vi "database_connection_write_dev_MQTT_no_database_array.vi"(6 "connection reference":T2, 7 "string":string="Raw.DMG_MORI_DMU_40_EVO", 8 "error in (no error)":errorcluster, 9 "data 2":dbl[](array[numeric]), 10 "Machine Data":T3={"Zload"="", "Yload"="", "Xload"="", "path_position"="", "Fovr"="", "SspeedOvr"="", "Program Name"="", "Program status"="", "Block of code being executed"="", "Line of code"="", "Machine availability"="", "Emergency status"="", "Controller mode"="", "Tool_id"="UNAVAILABLE"}, 11 "current time 2":timestamp format="%^<%Y-%m-%d %H:%M:%S%3u>T") -> (0 "connection reference out":T2, 3 "error out":errorcluster)   [LabVIEW 2017]
uses:
  <vilib>/addons/database/Connection.llb/Conn ObjectReference.ctl
  data_base_structure_V2.ctl
  data_base_structure.ctl
  controls/databse_structure.ctl
  <vilib>/addons/database/NI_Database_API.lvlib
panel:
  out "output cluster 2":cluster{string, "Machine availability":string}
  out "output cluster":T1
  out "Array":string[](array[string])=["timestamp", "available", "execution", "controller_mode", "spindle_load", "spindle_speed", "sspeedovr", "feed_rate", "fovr", "I_part", "J_part", "K_part", "Xpos_part", "Ypos_part", "Zpos_part", "Apos_machine", "Bpos_machine", "Xload", "Yload", "Zload", "Aload", "Bload", "tool_id", "program_number", "program_name", "block_code", "line_number", "estop", "accel_x_rms", "accel_y_rms", "accel_z_rms"]
  out "Program Name":string
  out "date/time string 2":string
  out "ISO-8601 UTC Formatted DateTime String":string
  out "error out 2":errorcluster
  in  "error in":errorcluster
  out "Timestamp":timestamp
  out "date/time string":string
  out "current time 3":timestamp
  out "resulting string 2":string
  out "Xload":string
  out "Machine availability":string
  out "resulting string":string
  out "output array 2":dbl[](array[numeric])
  out "size(s) 2":i32
  out "valueSent 2":string="14:19:17.238_"
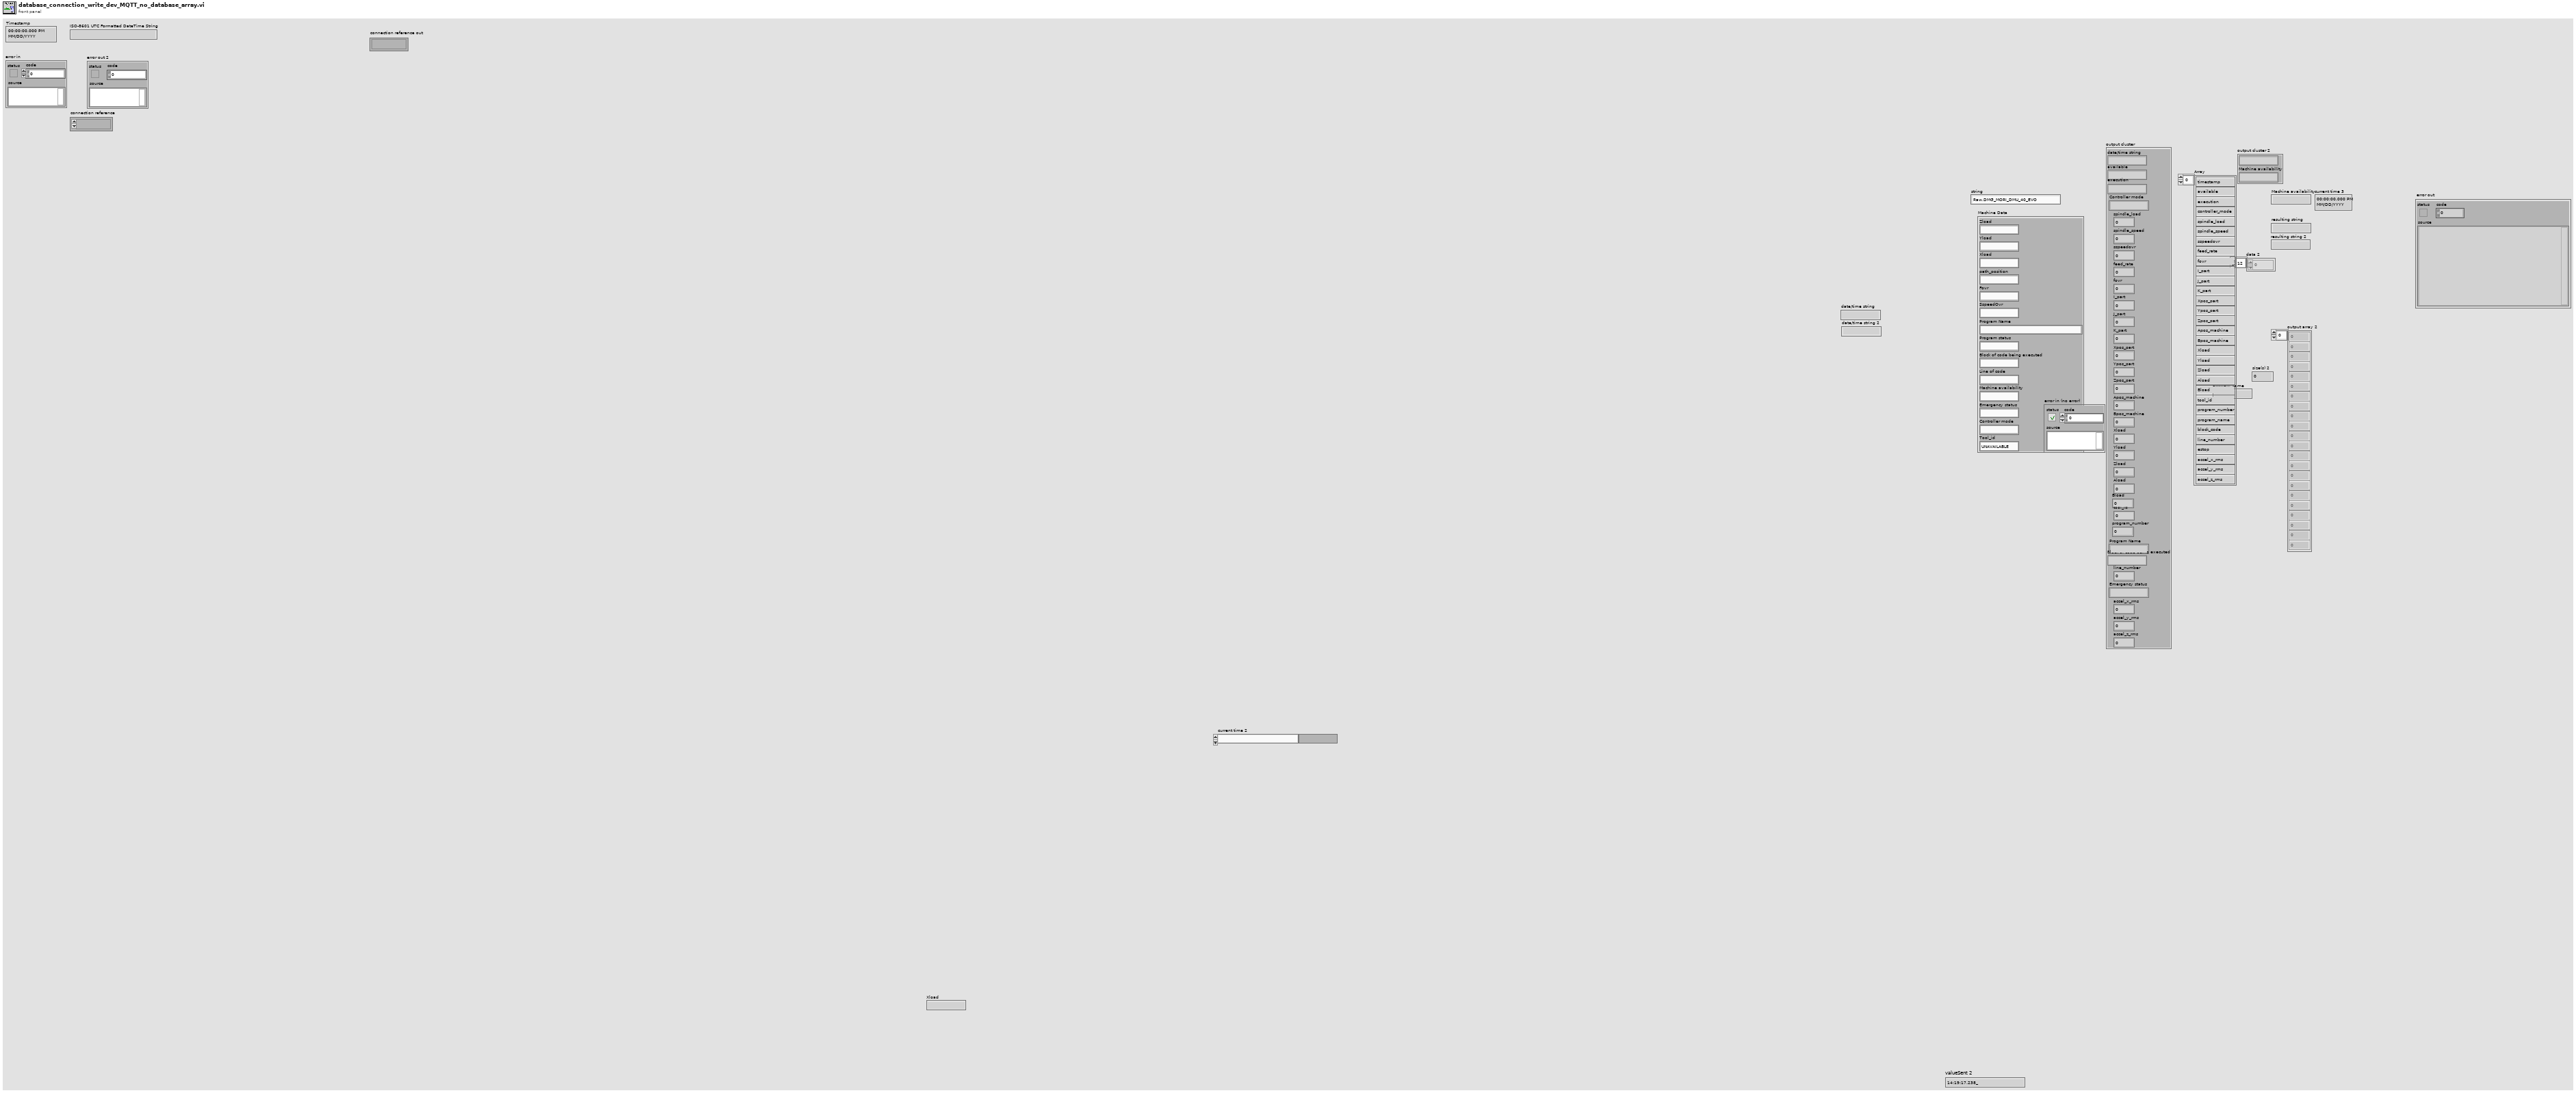
[diagram p1: front panel]
types:
  T1 = typedef "data_base_structure_V2.ctl" = cluster{"date/time string":string, "available":string, "Controller mode":string, "spindle_load":dbl, "spindle_speed":dbl, "sspeedovr":dbl, "feed_rate":dbl, "fovr":dbl, "I_part":dbl, "J_part":dbl, "K_part":dbl, "Xpos_part":dbl, "Ypos_part":dbl, "Zpos_part":dbl, "Apos_machine":dbl, "Bpos_machine":dbl, "Xload":dbl, "Yload":dbl, "Zload":dbl, "Aload":dbl, "Bload":dbl, "tool_id":dbl, "program_number":dbl, "Program Name":string, "Block of code being executed":string, "line_number":dbl, "Emergency status":string, "accel_x_rms":dbl, "accel_y_rms":dbl, "accel_z_rms":dbl, "execution":string}
  T2 = typedef "NI_Database_API.lvlib/Conn ObjectReference.ctl" = refnum<k1>
  T3 = cluster{"Zload":string, "Yload":string, "Xload":string, "path_position":string, "Fovr":string, "SspeedOvr":string, "Program Name":string, "Program status":string, "Block of code being executed":string, "Line of code":string, "Machine availability":string, "Emergency status":string, "Controller mode":string, "Tool_id":string}
  T4 = typedef "data_base_structure.ctl" = cluster{"available ":dbl, "controller_mode":string, "spindle_load":dbl, "spindle_speed ":dbl, "sspeedovr":dbl, "J_part":dbl, "K_part":dbl, "Xpos_part":dbl, "Ypos_part":dbl, "Zpos_part":dbl, "Apos_machine":dbl, "Bpos_machine":dbl, "Xload":dbl, "Yload":dbl, "Zload":dbl, "Aload":dbl, "Bload":dbl, "tool_id":dbl, "program_name":string, "block_code":string, "line_number":dbl, "estop":string, "accel_x_rms":dbl, "accel_y_rms":dbl, "accel_z_rms":dbl, "program_number":dbl, "timestamp":string, "feed_rate ":dbl, "fovr":dbl, "I_part ":dbl}
  T5 = cluster{"date/time string":string, "available":string, "execution":string, "Controller mode":string, "spindle_load":dbl, "spindle_speed":dbl, "sspeedovr":dbl, "feed_rate":dbl, "fovr":dbl, "I_part":dbl, "J_part":dbl, "K_part":dbl, "Xpos_part":dbl, "Ypos_part":dbl, "Zpos_part":dbl, "Apos_machine":dbl, "Bpos_machine":dbl, "Xload":dbl, "Yload":dbl, "Zload":dbl, "Aload":dbl, "Bload":dbl, "tool_id":dbl, "program_number":dbl, "Program Name":string, "Block of code being executed":string, "line_number":dbl, "Emergency status":string, "accel_x_rms":dbl, "accel_y_rms":dbl, "accel_z_rms":dbl}
  T6 = typedef "databse_structure.ctl" = cluster{"date/time string":string, "available":string, "execution":string, "Controller mode":string, "accel_z_rms":dbl, "accel_y_rms":dbl, "accel_x_rms":dbl, "Emergency status":string, "line_number":dbl, "Block of code being executed":string, "Program Name":string, "program_number":dbl, "tool_id":dbl, "Bload":dbl, "Aload":dbl, "Zload":dbl, "Yload":dbl, "Xload":dbl, "Bpos_machine":dbl, "Apos_machine":dbl, "Zpos_part":dbl, "Ypos_part":dbl, "Xpos_part":dbl, "K_part":dbl, "J_part":dbl, "I_part":dbl, "fovr":dbl, "feed_rate":dbl, "sspeedovr":dbl, "spindle_speed":dbl, "spindle_load":dbl}
  T7 = cluster{"data 2[0]":dbl, "data 2[1]":dbl, "data 2[2]":dbl, "data 2[3]":dbl, "data 2[4]":dbl, "data 2[5]":dbl, "data 2[6]":dbl, "data 2[7]":dbl, "data 2[8]":dbl, "data 2[9]":dbl, "data 2[10]":dbl, "data 2[11]":dbl, "data 2[12]":dbl, "data 2[13]":dbl, "data 2[14]":dbl, "data 2[15]":dbl, "data 2[16]":dbl, "data 2[17]":dbl, "data 2[18]":dbl, "data 2[19]":dbl, "data 2[20]":dbl, "data 2[21]":dbl}
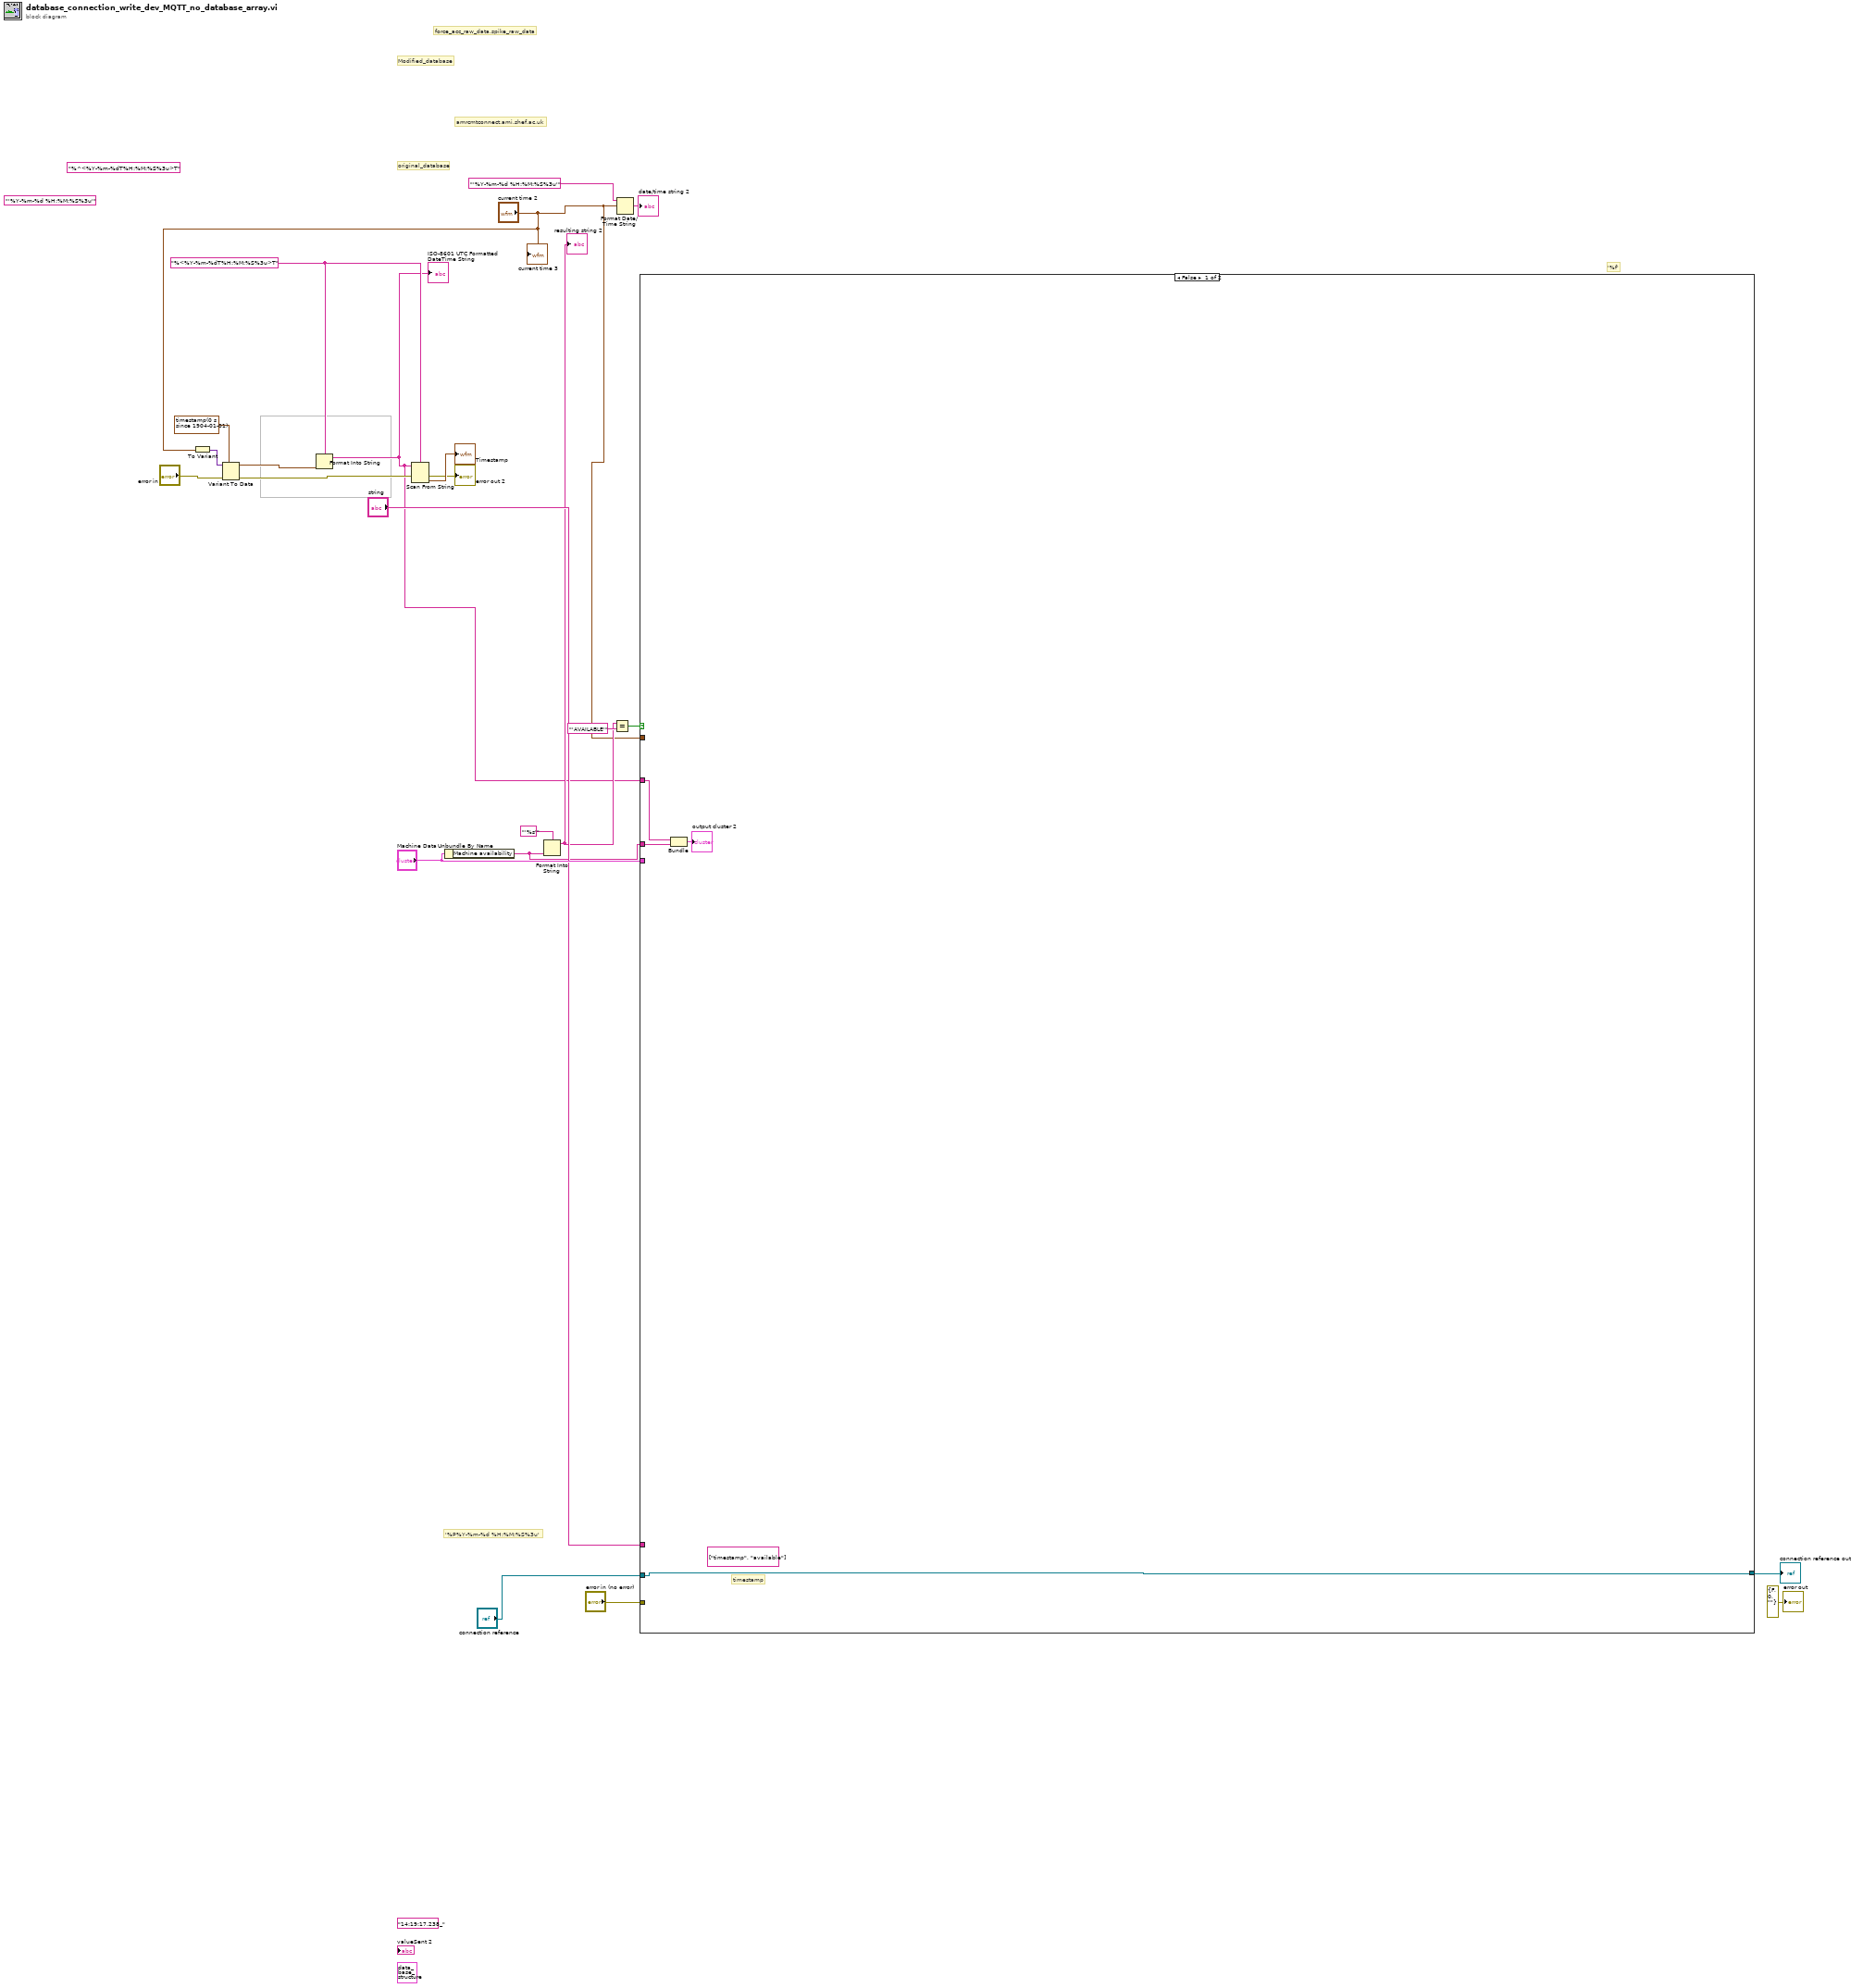
[diagram p0: block diagram]
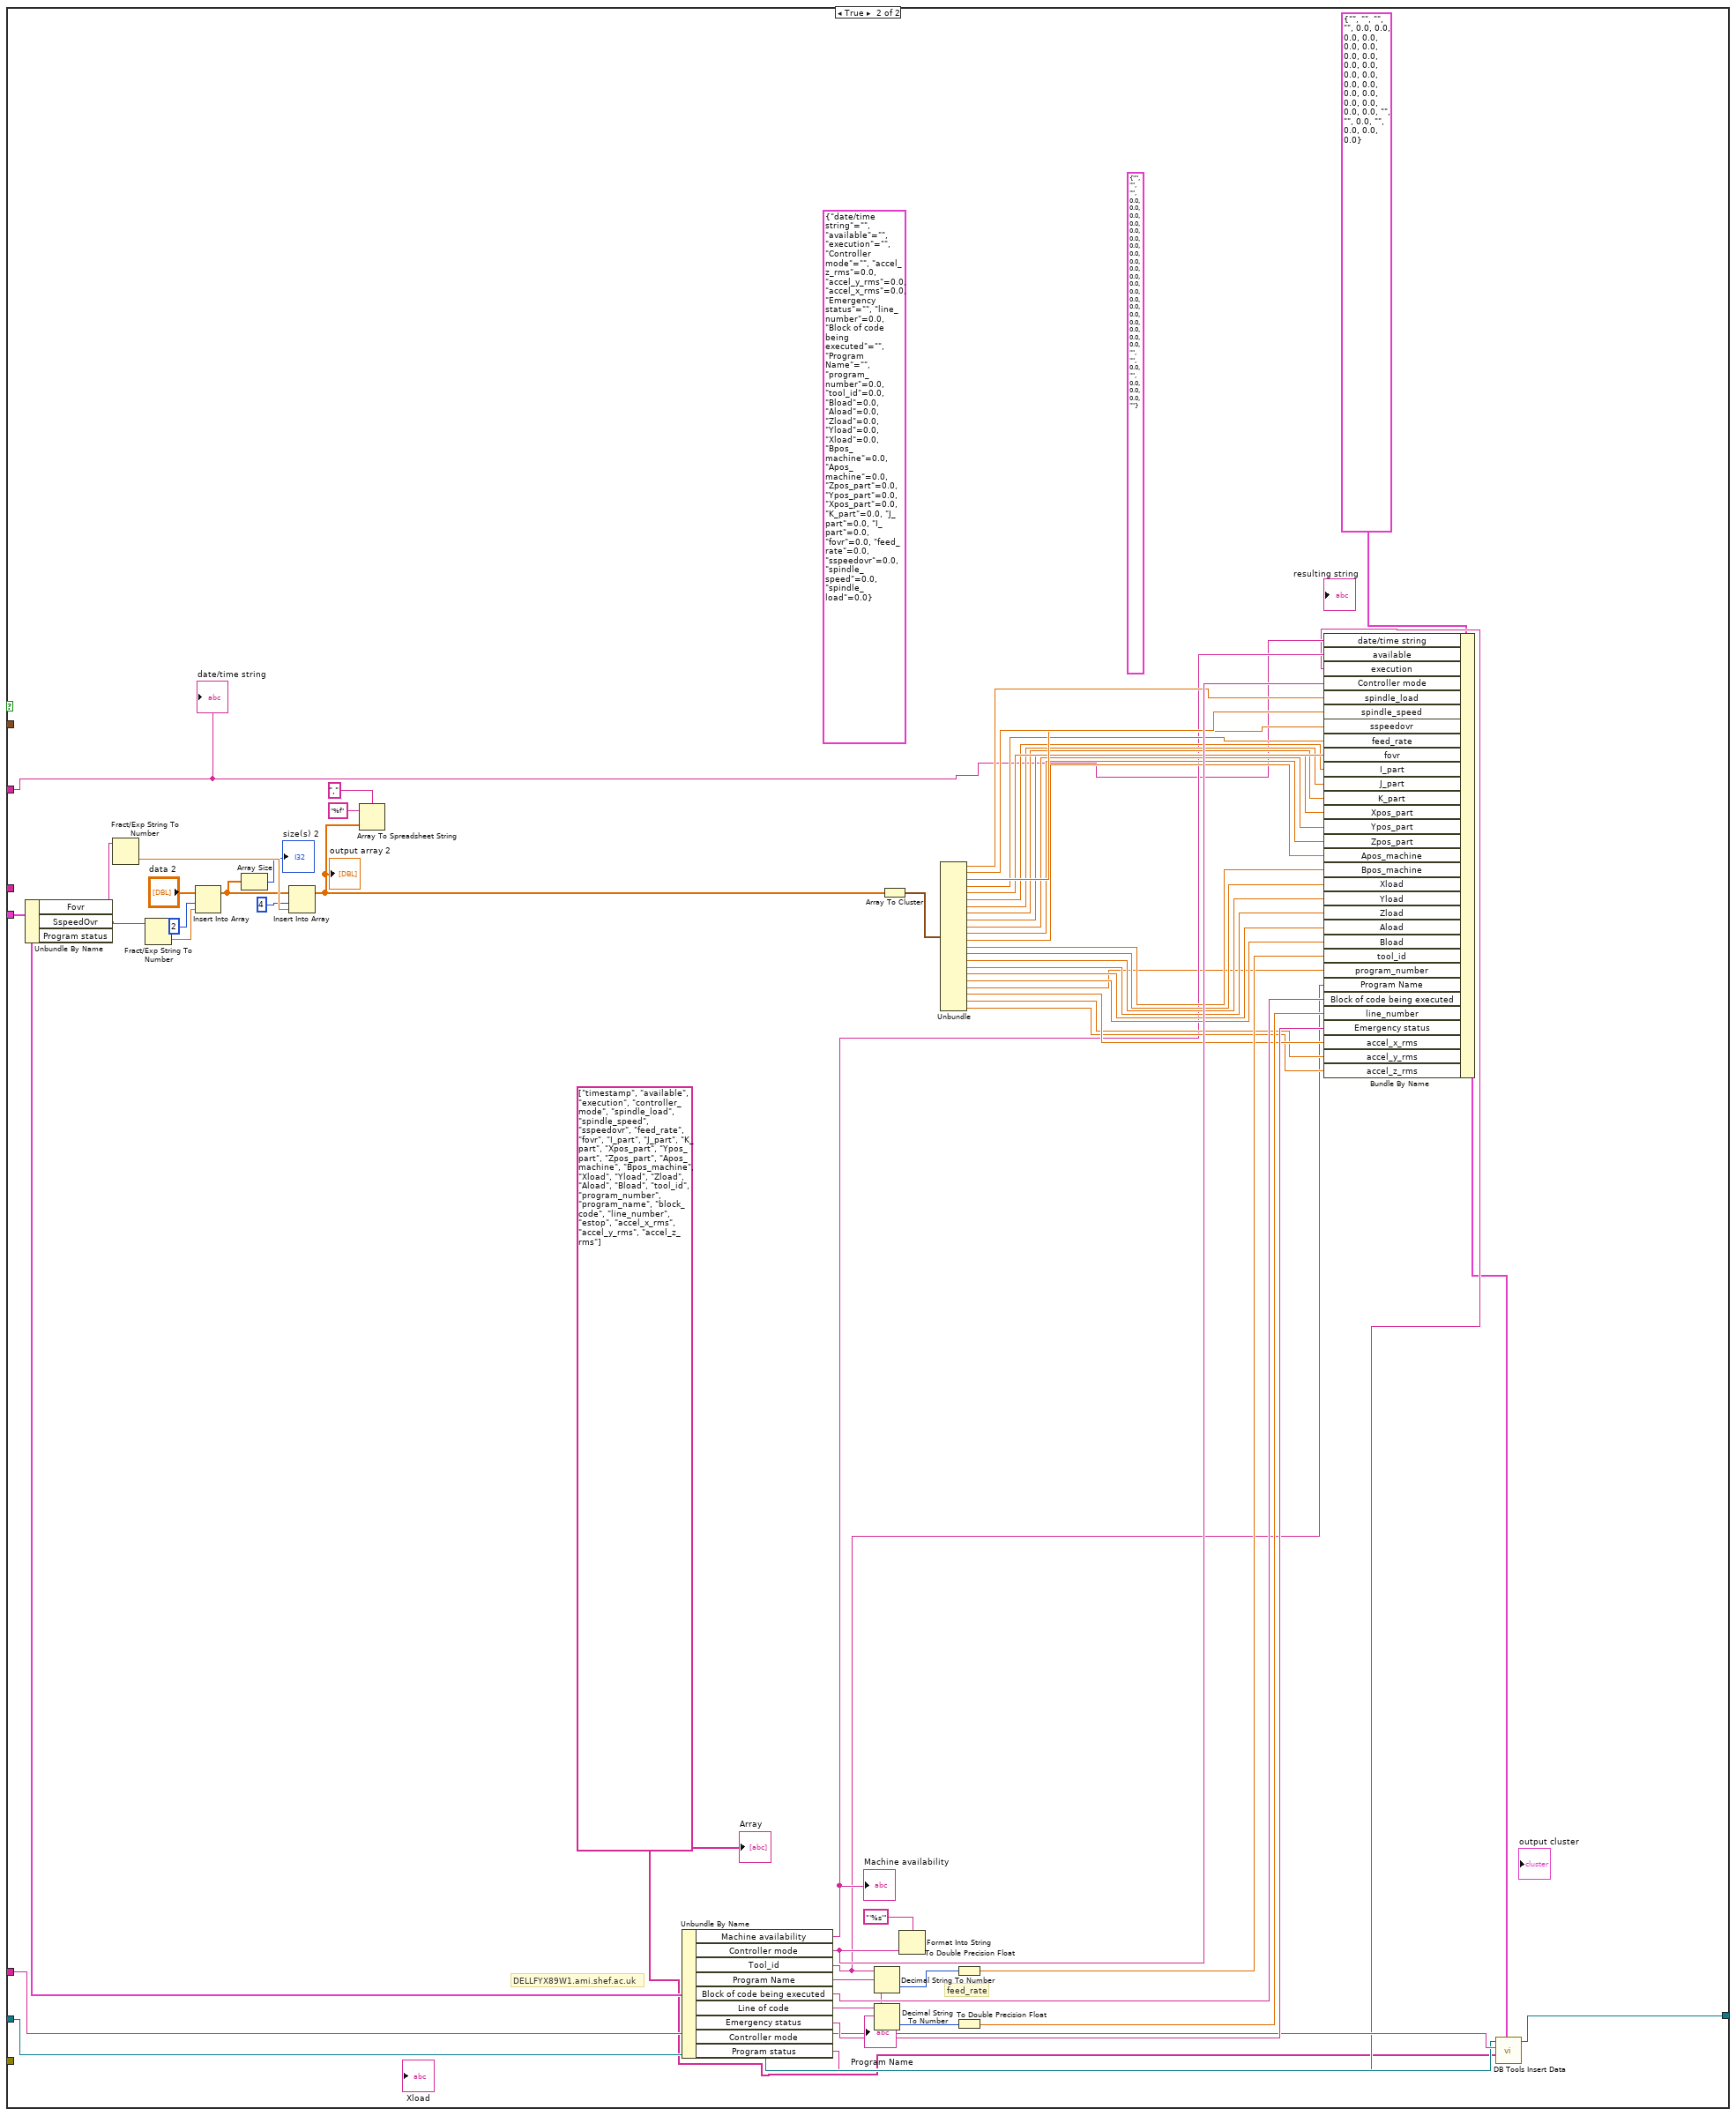
[diagram p2: hidden frame]
diagram:
  (unwired) "%^<%Y-%m-%dT%H:%M:%S%3u>T" ("format string")
  (unwired) "'%Y-%m-%d %H:%M:%S%3u'" ("time format string (%c)")
  w9 = "%<%Y-%m-%dT%H:%M:%S%3u>T" ("format string")
  (unwired) "14:19:17.238_" ("valueSent 2")
  (unwired) T4 {"available "=0.0, "controller_mode"="", "spindle_load"=0.0, "spindle_speed "=0.0, "sspeedovr"=0.0, "J_part"=0.0, "K_part"=0.0, "Xpos_part"=0.0, "Ypos_part"=0.0, "Zpos_part"=0.0, "Apos_machine"=0.0, "Bpos_machine"=0.0, "Xload"=0.0, "Yload"=0.0, "Zload"=0.0, "Aload"=0.0, "Bload"=0.0, "tool_id"=0.0, "program_name"="", "block_code"="", "line_number"=0.0, "estop"="", "accel_x_rms"=0.0, "accel_y_rms"=0.0, "accel_z_rms"=0.0, "program_number"=0.0, "timestamp"="", "feed_rate "=0.0, "fovr"=0.0, "I_part "=0.0} ("Cluster")
  # "'%P%Y-%m-%d %H:%M:%S%3u'"
  # "'%f'"
  # "original_database"
  # "force_acc_raw_data,spike_raw_data"
  # "Modified_database"
  # "amrcmtconnect.ami.shef.ac.uk"
  n1 = To Variant(anything="current time 2") -> (Variant=w14:variant)
  n2 = Variant To Data(error in="error in", type=timestamp(0 s since 1904-01-01) ("time stamp"), Variant=w14) -> (data=w8:timestamp, error out=w11:errorcluster)
  n3 = Format Into String(format string=w9, w8) -> (resulting string=w6:string)  [unwired: 2 in, 1 out]
  "ISO-8601 UTC Formatted DateTime String" <- w6
  n4 = Scan From String(format string=w9, input string=w6, error in=w11) -> (error out=→"error out 2":errorcluster, output 1=→"Timestamp":timestamp)  [unwired: 2 in, 2 out]
  n5 = Unbundle By Name("Machine Data") -> ("Machine availability"=w2:string)
  n6 = Format Into String(format string="'%s'", w2) -> (resulting string=w16:string)  [unwired: 2 in, 1 out]
  "resulting string 2" <- w16
  n7 = Equal?(x=w16, y="'AVAILABLE'") -> (x = y?=w19:bool)
  n8 = Format Date/Time String(time format string (%c)="'%Y-%m-%d %H:%M:%S%3u'", seconds (now)="current time 2") -> (date/time string=→"date/time string 2":string)  [unwired: 1 in]
  n9 = case shown="False" w19 {
    tunnel: "Machine Data" -> [_ w39]
    tunnel: "error in (no error)" -> [_ _]
    tunnel: "string" -> [_ w38]
    tunnel: w2 -> [w26 _]
    tunnel: "current time 2" -> [_ _]
    tunnel: w6 -> [w27 w37]
    tunnel: "connection reference" -> [w25 w36]
    tunnel: [w25 w35] -> w3
    frame False {
      (unwired) string[] ["timestamp", "available"]
      # "timestamp"
      n10 = Bundle(w27, "Machine availability"=w26) -> (→"output cluster 2":cluster{string, "Machine availability":string})  [unwired: 1 in]
    }
    frame True {
      (unwired) T6 {"date/time string"="", "available"="", "execution"="", "Controller mode"="", "accel_z_rms"=0.0, "accel_y_rms"=0.0, "accel_x_rms"=0.0, "Emergency status"="", "line_number"=0.0, "Block of code being executed"="", "Program Name"="", "program_number"=0.0, "tool_id"=0.0, "Bload"=0.0, "Aload"=0.0, "Zload"=0.0, "Yload"=0.0, "Xload"=0.0, "Bpos_machine"=0.0, "Apos_machine"=0.0, "Zpos_part"=0.0, "Ypos_part"=0.0, "Xpos_part"=0.0, "K_part"=0.0, "J_part"=0.0, "I_part"=0.0, "fovr"=0.0, "feed_rate"=0.0, "sspeedovr"=0.0, "spindle_speed"=0.0, "spindle_load"=0.0}
      w30 = string[] ["timestamp", "available", "execution", "controller_mode", "spindle_load", "spindle_speed", "sspeedovr", "feed_rate", "fovr", "I_part", "J_part", "K_part", "Xpos_part", "Ypos_part", "Zpos_part", "Apos_machine", "Bpos_machine", "Xload", "Yload", "Zload", "Aload", "Bload", "tool_id", "program_number", "program_name", "block_code", "line_number", "estop", "accel_x_rms", "accel_y_rms", "accel_z_rms"]
      (unwired) T1 {"date/time string"="", "available"="", "Controller mode"="", "spindle_load"=0.0, "spindle_speed"=0.0, "sspeedovr"=0.0, "feed_rate"=0.0, "fovr"=0.0, "I_part"=0.0, "J_part"=0.0, "K_part"=0.0, "Xpos_part"=0.0, "Ypos_part"=0.0, "Zpos_part"=0.0, "Apos_machine"=0.0, "Bpos_machine"=0.0, "Xload"=0.0, "Yload"=0.0, "Zload"=0.0, "Aload"=0.0, "Bload"=0.0, "tool_id"=0.0, "program_number"=0.0, "Program Name"="", "Block of code being executed"="", "line_number"=0.0, "Emergency status"="", "accel_x_rms"=0.0, "accel_y_rms"=0.0, "accel_z_rms"=0.0, "execution"=""} ("cluster")
      # "feed_rate"
      # "DELLFYX89W1.ami.shef.ac.uk"
      n11 = Unbundle By Name(w39) -> ("Fovr"=w75:string, "SspeedOvr"=w80:string)  [unwired: 1 out]
      n12 = Fract/Exp String To Number(string=w75) -> (number=w77:dbl)  [unwired: 3 in, 1 out]
      n13 = Fract/Exp String To Number(string=w80) -> (number=w79:dbl)  [unwired: 3 in, 1 out]
      n14 = Insert Into Array(array="data 2", index=2, new element=w79) -> (w73:dbl[])
      n15 = Array Size(array=w73) -> (size(s)=→"size(s) 2":i32)
      n16 = Insert Into Array(array=w73, index=4, new element=w77) -> (w68:dbl[])
      "output array 2" <- w68
      n17 = Array To Spreadsheet String(delimiter (Tab)=",", array=w68, 3:"%f" ("format string")) -> ()  [unwired: 1 out]
      n18 = Unbundle By Name(w39) -> ("Machine availability"=w40:string, "Controller mode"=w66:string, "Tool_id"=w32:string, "Program Name"=→"Program Name":string, "Block of code being executed"=w46:string, "Line of code"=w71:string, "Emergency status"=w44:string, "Program status"=w31:string)  [unwired: 1 out]
      "Machine availability" <- w40
      n19 = Decimal String To Number(string=w32) -> (number=w72:i32)  [unwired: 2 in, 1 out]
      n20 = Decimal String To Number(string=w71) -> (number=w70:i32)  [unwired: 2 in, 1 out]
      n21 = Array To Cluster(array=w68) -> (cluster=w67:T7)
      n22 = Format Into String(format string="'%s'", w66) -> ()  [unwired: 2 in, 2 out]
      n23 = Unbundle(w67) -> ("data 2[0]"=w65:dbl, "data 2[1]"=w64:dbl, "data 2[2]"=w63:dbl, "data 2[3]"=w62:dbl, "data 2[4]"=w61:dbl, "data 2[5]"=w60:dbl, "data 2[6]"=w59:dbl, "data 2[7]"=w58:dbl, "data 2[8]"=w57:dbl, "data 2[9]"=w56:dbl, "data 2[10]"=w55:dbl, "data 2[11]"=w54:dbl, "data 2[12]"=w53:dbl, "data 2[13]"=w52:dbl, "data 2[14]"=w51:dbl, "data 2[15]"=w50:dbl, "data 2[16]"=w49:dbl, "data 2[17]"=w48:dbl, "data 2[18]"=w33:dbl, "data 2[19]"=w43:dbl, "data 2[20]"=w42:dbl, "data 2[21]"=w41:dbl)
      n24 = To Double Precision Float(number=w72) -> (double precision float=w47:dbl)
      n25 = To Double Precision Float(number=w70) -> (double precision float=w45:dbl)
      n26 = Bundle By Name(cluster=T5 {"date/time string"="", "available"="", "execution"="", "Controller mode"="", "spindle_load"=0.0, "spindle_speed"=0.0, "sspeedovr"=0.0, "feed_rate"=0.0, "fovr"=0.0, "I_part"=0.0, "J_part"=0.0, "K_part"=0.0, "Xpos_part"=0.0, "Ypos_part"=0.0, "Zpos_part"=0.0, "Apos_machine"=0.0, "Bpos_machine"=0.0, "Xload"=0.0, "Yload"=0.0, "Zload"=0.0, "Aload"=0.0, "Bload"=0.0, "tool_id"=0.0, "program_number"=0.0, "Program Name"="", "Block of code being executed"="", "line_number"=0.0, "Emergency status"="", "accel_x_rms"=0.0, "accel_y_rms"=0.0, "accel_z_rms"=0.0}, "date/time string"=w37, "available"=w40, "execution"=w31, "Controller mode"=w66, "spindle_load"=w65, "spindle_speed"=w64, "sspeedovr"=w63, "feed_rate"=w62, "fovr"=w61, "I_part"=w60, "J_part"=w59, "K_part"=w58, "Xpos_part"=w57, "Ypos_part"=w56, "Zpos_part"=w55, "Apos_machine"=w54, "Bpos_machine"=w53, "Xload"=w52, "Yload"=w51, "Zload"=w50, "Aload"=w49, "Bload"=w48, "tool_id"=w47, "program_number"=w33, "Program Name"=w32, "Block of code being executed"=w46, "line_number"=w45, "Emergency status"=w44, "accel_x_rms"=w43, "accel_y_rms"=w42, "accel_z_rms"=w41) -> (w29:T5)
      n27 = call <vilib>:"DB Tools Insert Data.vi"("data"=w29, "columns"=w30, "table"=w38, "connection reference"=w36) -> ("connection reference out"=w35:T2)  [unwired: 6 in, 1 out]
      "date/time string" <- w37
      "Array" <- w30
    }
  }
  "connection reference out" <- w3
  "error out" <- errorcluster {"status"=FALSE, "code"=0, "source"=""} ("error out")
  "current time 3" <- "current time 2"
